vi "Publish Report.vi"(8 "error in (no error)":errorcluster, 11 "ResultProcessor in":refnum<class "ResultProcessor.lvclass">) -> (0 "error out":errorcluster, 3 "ResultProcessor out":refnum<class "ResultProcessor.lvclass">)   [LabVIEW 2015, in "ResultProcessor.lvclass"]
doc: "This VI will save the report in all of the configured formats."
uses:
  ResultProcessor.lvclass
  CommandQueueDataType.ctl
  Report Information/Report Information.lvclass
  Result/Result.lvclass
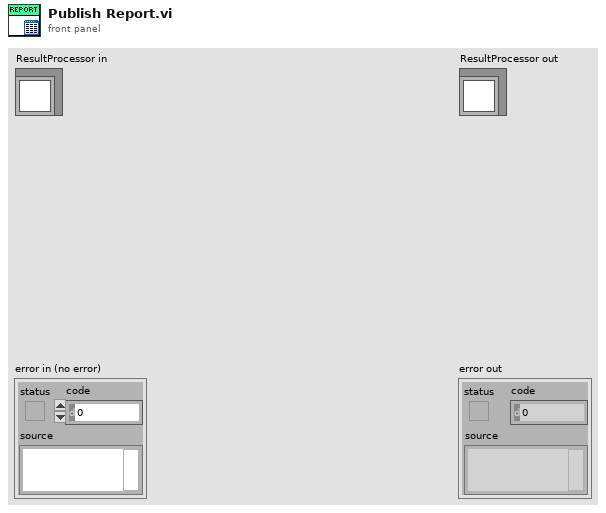
[diagram p1: front panel]
types:
  T1 = typedef "ResultProcessor.lvclass/CommandQueueDataType.ctl" = cluster{"Command":enum16{"New Report", "Add Result", "Publish Report", "Shutdown", "Add DUT Information", "Add Station Information", "Add Report Information", "Add Test Information"}, "Report Information.lvclass":refnum<class "Report Information.lvclass">, "Result.lvclass":refnum<class "Result.lvclass">}
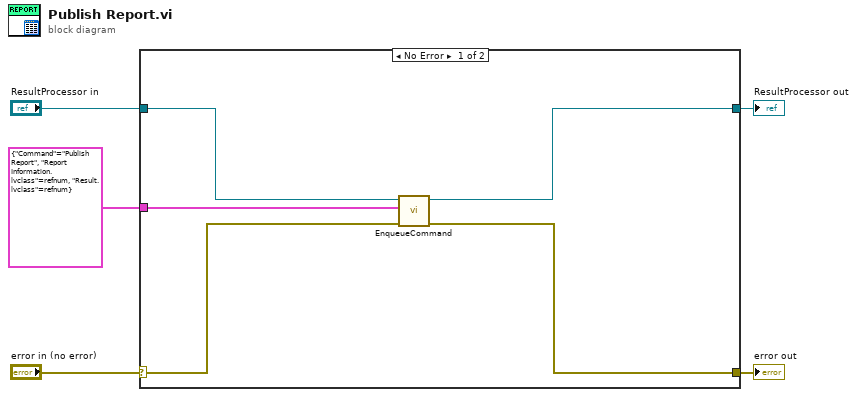
[diagram p0: block diagram]
diagram:
  n1 = case shown="No Error" "error in (no error)" {
    selector: "error in (no error)" -> [w9 w12]
    tunnel: [w8 w12] -> w3
    tunnel: [w7 w11] -> w2
    tunnel: "ResultProcessor in" -> [w10 w11]
    tunnel: T1 {"Command"=enum."Publish Report", "Report Information.lvclass"=refnum, "Result.lvclass"=refnum} ("element") -> [w6 _]
    frame No Error {
      n2 = call "EnqueueCommand.vi"("error in (no error)"=w9, "element"=w6, "ResultProcessor in"=w10) -> ("error out"=w8:errorcluster, "ResultProcessor out"=w7:refnum<class "ResultProcessor.lvclass">)  [unwired: 7 in]
    }
    frame Error {
    }
  }
  "error out" <- w3
  "ResultProcessor out" <- w2
